vi "End.vi"(8 "error in (no error)":errorcluster, 11 "Channel in":refnum<class "Channel.lvclass">) -> (0 "error out":errorcluster, 3 "Channel out":refnum<class "Channel.lvclass">)   [LabVIEW 2018, in "Channel.lvclass"]
uses:
  Channel.lvclass
  Channel.lvclass/Channel.ctl
  RxTx/RxTx.lvclass
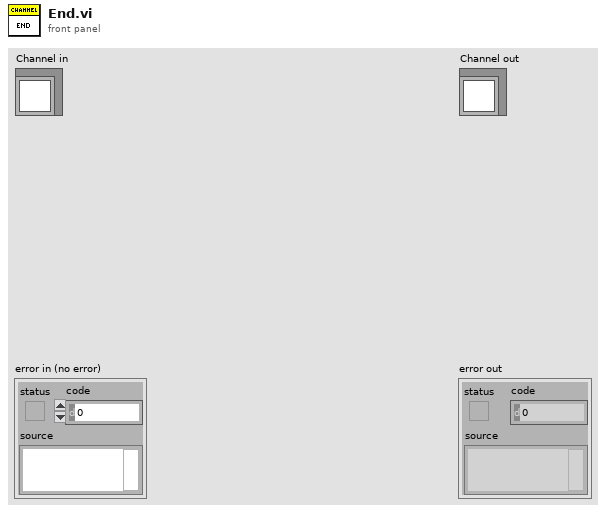
[diagram p1: front panel]
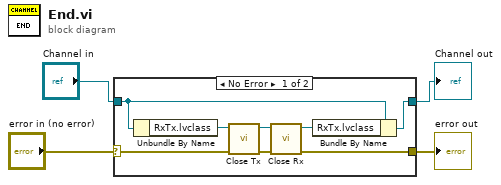
[diagram p0: block diagram]
diagram:
  n1 = case shown="No Error" "error in (no error)" {
    selector: "error in (no error)" -> [w6 w14]
    tunnel: [w10 w14] -> w3
    tunnel: [w11 w13] -> w1
    tunnel: "Channel in" -> [w12 w13]
    frame No Error {
      n2 = Unbundle By Name(w12) -> ("RxTx.lvclass"=w7:refnum<class "RxTx.lvclass">)
      n3 = call "Close Tx.vi"("error in (no error)"=w6, "RxTx in"=w7) -> ("error out"=w5:errorcluster, "RxTx out"=w8:refnum<class "RxTx.lvclass">)  [unwired: 8 in]
      n4 = call "Close Rx.vi"("error in (no error)"=w5, "RxTx in"=w8) -> ("error out"=w10:errorcluster, "RxTx out"=w9:refnum<class "RxTx.lvclass">)  [unwired: 8 in]
      n5 = Bundle By Name(cluster=w12, "RxTx.lvclass"=w9) -> (w11:refnum<class "Channel.lvclass">)
    }
    frame Error {
    }
  }
  "error out" <- w3
  "Channel out" <- w1
